vi "get_status.vi"(8 "error in (no error)":errorcluster, 11 "Pistofono in":refnum<class "Pistofono.lvclass">) -> (0 "error out":errorcluster, 2 "status":cluster{"status":bool, "source":string}={"status"=TRUE, "source"=""}, 3 "Pistofono out":refnum<class "Pistofono.lvclass">)   [LabVIEW 2019, in "Pistofono.lvclass"]
uses:
  Pistofono.lvclass
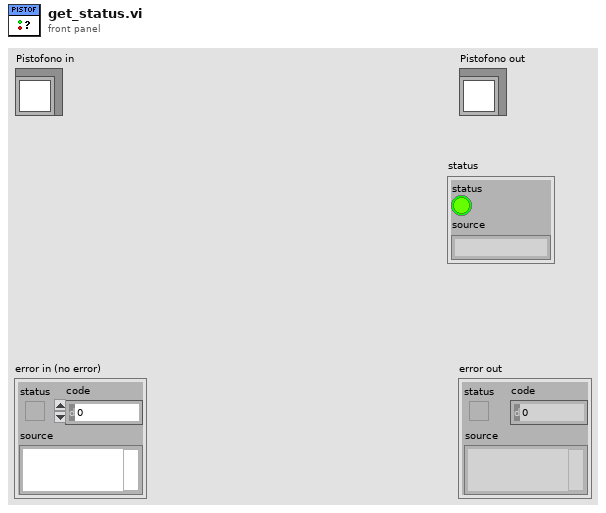
[diagram p1: front panel]
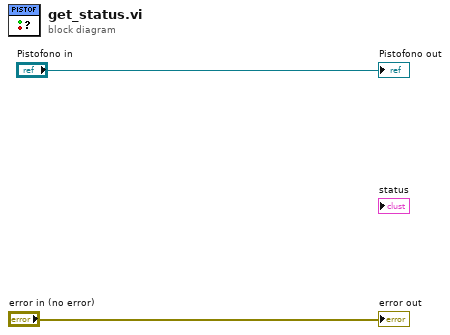
[diagram p0: block diagram]
diagram:
  "error out" <- "error in (no error)"
  "Pistofono out" <- "Pistofono in"
